vi "Schedule.vi"() -> ()   [LabVIEW 2016]
panel:
  in  "Previous Button":bool
  # "Schedule"
  # "The seven day week consists of five and half days schedule for working nominal tasks and a contiguous 1.5 days off.  That doesn't necessarily mean the crew do no work during that 1.5 days, just that they aren't scheduled for tasks other than mandatory things like exercise.\n\nA 24 hour day is composed of 8.5 hours allotted for sleep. 6.5 hours allotted to scheduled work tasks, 2.5 hours schedule for required exercise, 1 hour scheduled for lunch.  There is also time allotted for daily planning conferences with the ground, work preparation time (time to read procedures and gather tools), and plan familiarization time (time to review the day's schedule).  And then pre-sleep and post-sleep time during which hygiene activities, dinner, and breakfast are completed."
  # "Here are two typical daily plans for an astronaut aboard the International Space Station (ISS):\n \nDay 1\n06:00 GMT  wake up  personal time\n07:30 Discuss today's work with the ground\n07:45 Daily tasks – maintenance, payloads etc.\n09:45 Exercise on Bike 1hr\n10:45 Exercise rope strength training 1 hr (Medical)\n11:45 Strength training 1:20m\n13:00 Lunch\n14:00 EVA Suit maintenance\n14:30 Prep for a PAO\n14:40 PAO (Public Affairs activities) 20m\n15:00 ATV transfer operations\n16:30 PMC (Private Medical Conference with the ground)\n17:10 PPC (Private Psychological Conference)\n17:40 ATV transfer operations\n18:35 prep for next day\n19:05 Discuss day's work with the ground\n19:30 personal time before sleep\n21:30 Sleep"
  # "Day 2\n06:00 GMT  wake up  personal time\n07:30 Discuss today's work with the ground\n08:15 Install Alignment Guides for Flammable Liquids Cabinet\n08:25 ATV Transfer\n09:50 Spinal Elongation Microgravity Experiment\n11:30 Load Platform Serial Network Flow Monitor Scientific Hardware Cabinet\n11:45 Switch Load Scientific Experiment\n12:00 Binary Colloidal Alloy Experiment\n12:20 Conference with ground about storage of supplies\n12:40 Switch Load Biological Research System Experiment\n12:55 Lunch\n13:55 ATV Transfer\n15:15 Strength Training\n16:45 ATV Transfer\n16:55 Treadmill Exercise\n18:15 Prepare for Next Day's Work\n18:45 Discuss today's work with ground\n19:10 Prepare for Next Day's Work\n19:30 Personal time before going to sleep\n21:20 Spinal Elongation Experiment\n21:25 Binary Colloidal Alloy Experiment\n21:30 Sleep"
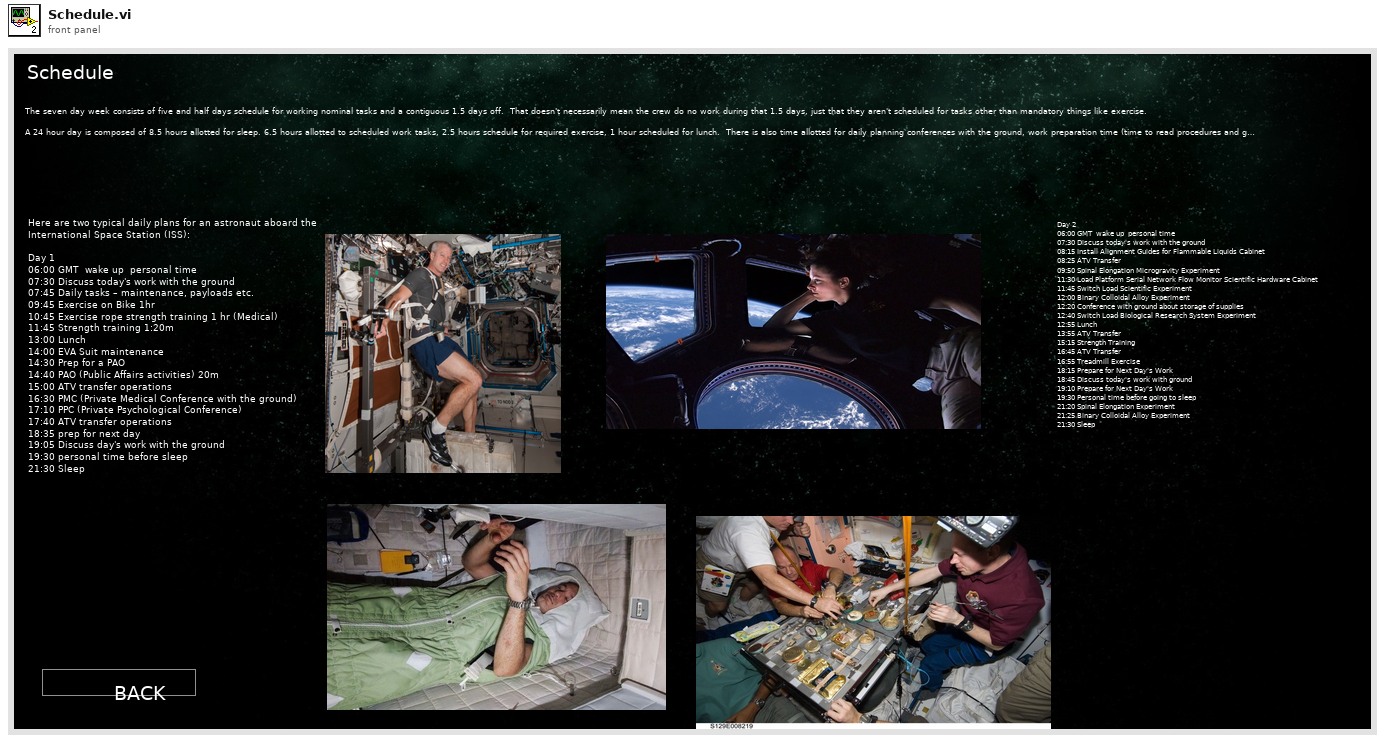
[diagram p1: front panel]
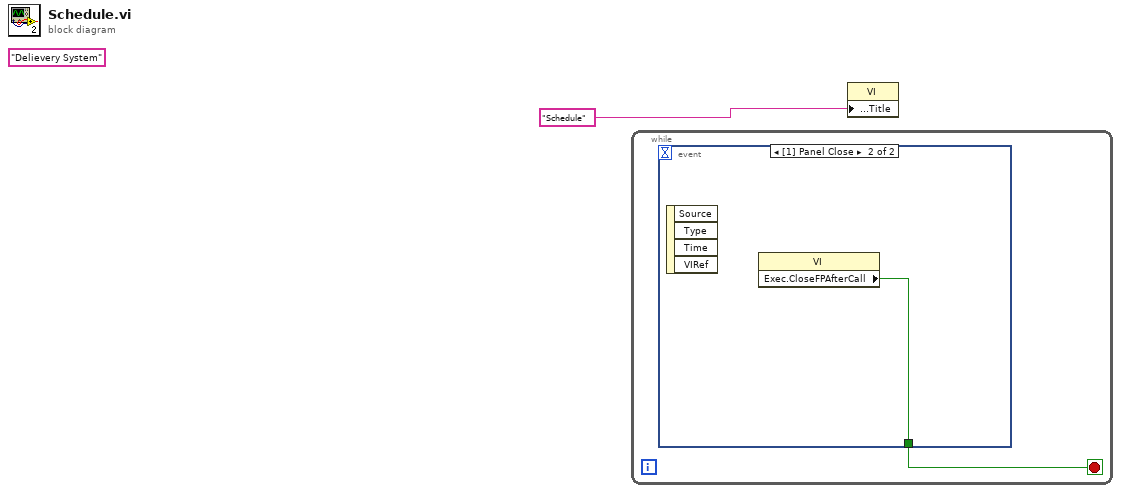
[diagram p0: block diagram]
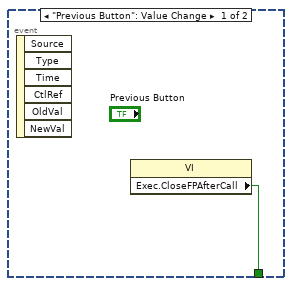
[diagram p2: hidden frame]
diagram:
  (unwired) "Delievery System" ("Front Panel Window:Title")
  n1 = while {
    stop <- w2 stop-if-true
    n2 = event shown="[1] Panel Close" {
      selector: _ -> [_ _]
      dyn-events: _ -> [_ _]
      timeout: _ -> [_ _]
      tunnel: [w3 w4] -> w2
      event "Previous Button": Value Change {
        n3 = event-data() -> ()  [unwired: 1 in, 6 out]
        n4 = property class="VI"() -> ("Exec.CloseFPAfterCall"=w3:bool)  [unwired: 2 in, 2 out]
      }
      event Panel Close {
        n5 = event-data() -> ()  [unwired: 1 in, 4 out]
        n6 = property class="VI"() -> ("Exec.CloseFPAfterCall"=w4:bool)  [unwired: 2 in, 2 out]
      }
    }
  }
  n7 = property class="VI"("Front Panel.Title"="Schedule" ("Front Panel Window:Title")) -> ()  [unwired: 2 in, 2 out]
